vi "lookup_node_by_id.vi"(10 "node_id":refnum<class "ID.lvclass">, 11 "graph":refnum<class "Graph.lvclass">) -> (1 "node":refnum<class "Node.lvclass">, 2 "node not found?":bool)   [LabVIEW 2020, in "graph.lvlib" / "Graph.lvclass"]
uses:
  Graph.lvclass
  ID/ID.lvclass
  Node/Node.lvclass
  Graph.lvclass/Graph.ctl
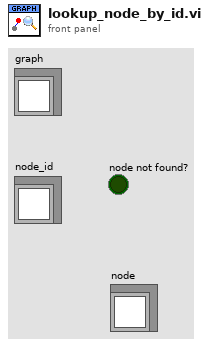
[diagram p1: front panel]
types:
  T1 = map{refnum<class "ID.lvclass">, refnum<class "Node.lvclass">}
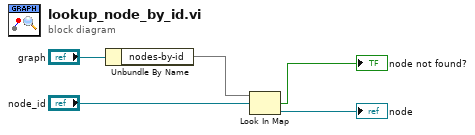
[diagram p0: block diagram]
diagram:
  n1 = Unbundle By Name("graph") -> ("nodes-by-id"=w1:T1)
  n2 = Look In Map(map=w1, key="node_id") -> (key not found?=→"node not found?":bool, value=→"node":refnum<class "Node.lvclass">)  [unwired: 1 in]
